vi "RSNRPZ Fast Zero.vi"(8 "error in (no error)":errorcluster, 11 "VISA session":refnum<visa-resource-name> caption="VISA resource name") -> (0 "error out":errorcluster, 3 "dup VISA session":refnum<visa-resource-name> caption="VISA resource name")   [LabVIEW 2010]
doc: "This VI performs fast zeroing, but can be called only in the sensor's Trace mode and Statistics modes. In any other measurement mode, the error message NRPERROR_CALZERO is output. Even though the execution time is shorter than that for standard zeroing by a factor of 100 or more, measurement accuracy is not affected. Fast zeroing is available for the entire frequency range.\n\nRemote-control command(s):\nCAL:ZERO:FAST:AUTO"
uses:
  rsnrpz_32.dll
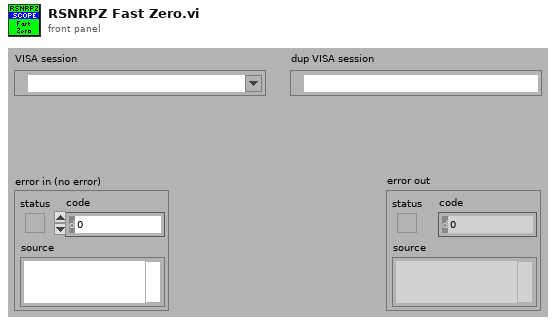
[diagram p1: front panel]
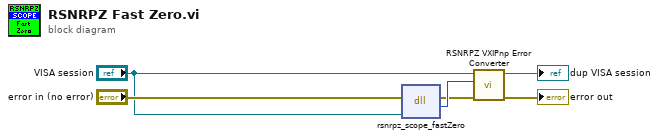
[diagram p0: block diagram]
diagram:
  n1 = dll-call lib="rsnrpz_32.dll" fn="rsnrpz_scope_fastZero"(error in="error in (no error)", "Instrument Handle"="VISA session") -> (error out=w5:errorcluster, "Status"=w6:i32)  [unwired: 3 in, 1 out]
  n2 = call <instrlib>:"RSNRPZ VXIPnp Error Converter.vi"("error in"=w5, "VXIPnp error code"=w6, "VISA session"="VISA session") -> ("error out"=→"error out":errorcluster, "dup VISA session"=→"dup VISA session":refnum<visa-resource-name>)  [unwired: 7 in]
